vi "Show Compatibility Warnings.vi"(8 "Error In":errorcluster, 9 "Can Continue?":bool, 10 "Warnings":T1[](array[typedef]), 11 "Install LV Data":T2={"SSH Session"=refnum, "Status Log"="", "Detailed Log"="", "Credentials"={"Hostname or IP"="192.168.7.2", "Username"="root", "Password"=""}, "Target Info"={"OS Version"="", "CPU"="", "Systemd Version"="", "Internet Access"=FALSE, "Device Type"="", "LV Installed Ver"="", "LV Available Ver"="", "LV Upgrade Available"=FALSE, "Hostname"="", "NIC Info"=[]}, "Reboot Required?"=FALSE}) -> (0 "Error Out":errorcluster, 1 "Continue?":bool, 2 "Warnings":T1[](array[typedef]), 3 "Install LV Data":T2={"SSH Session"=refnum, "Status Log"="", "Detailed Log"="", "Credentials"={"Hostname or IP"="192.168.7.2", "Username"="root", "Password"=""}, "Target Info"={"OS Version"="", "CPU"="", "Systemd Version"="", "Internet Access"=FALSE, "Device Type"="", "LV Installed Ver"="", "LV Available Ver"="", "LV Upgrade Available"=FALSE, "Hostname"="", "NIC Info"=[]}, "Reboot Required?"=FALSE})   [LabVIEW 2011, in "LMH-LINX.lvlib"]
uses:
  LMH-LINX.lvlib
  Target Compatibility Warnings.ctl
  User Warning.ctl
  Install LV Data.ctl
  C:/Users/samkristoff/Desktop/Builds/2016_01_27/build/LabVIEW/vi.lib/MakerHub/LINX/Resources/Renci.SshNet.dll
  Resources/Renci.SshNet.dll
  Target Info.ctl
  NIC Info.ctl
  NIC Mode.ctl
  Status FGV States.ctl
  <vilib>/Platform/browser.llb/Open URL in Default Browser (string).vi
  <vilib>/MakerHub/Toolbox/LMH-Toolbox.lvlib
panel:
  in  "Fix It":bool
  in  "Help":bool
  out "Warning Number":string
  in  "Next":bool
  in  "Previous":bool
  out "User Warnings Dialog":T6[](array[typedef])
  out "Title":string
  out "Main Text":string
  in  "Continue":bool
  in  "Cancel":bool
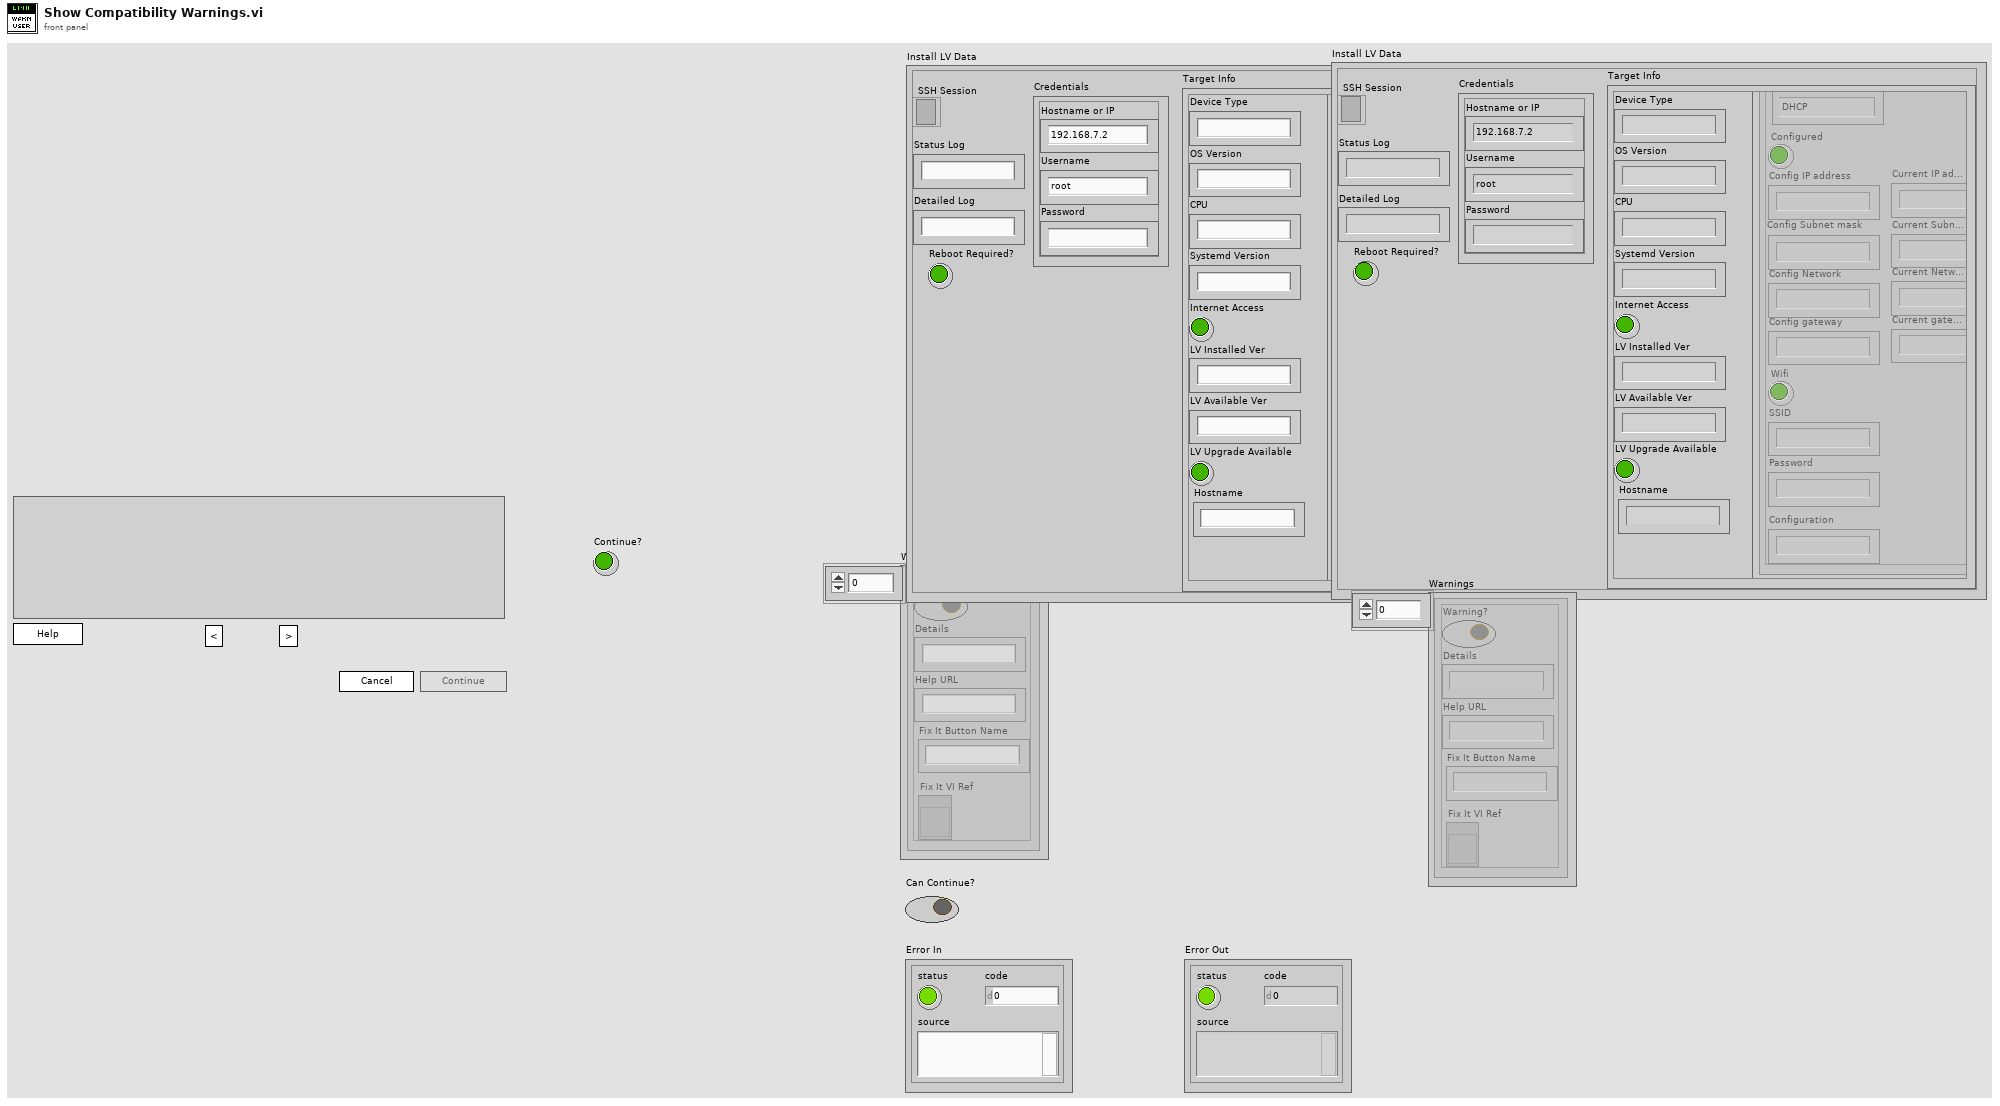
[diagram p1: front panel]
types:
  T1 = typedef "LMH-LINX.lvlib/Target Compatibility Warnings.ctl" = cluster{"Warning?":bool, "Details":string, "Help URL":string, "Fix It Button Name":string, "Fix It VI Ref":refnum<vi>}
  T2 = typedef "LMH-LINX.lvlib/Install LV Data.ctl" = cluster{"SSH Session":refnum<k24>, "Status Log":string, "Detailed Log":string, "Credentials":cluster{"Hostname or IP":string, "Username":string, "Password":string}, "Target Info":T3, "Reboot Required?":bool}
  T3 = typedef "LMH-LINX.lvlib/Target Info.ctl" = cluster{"OS Version":string, "CPU":string, "Systemd Version":string, "Internet Access":bool, "Device Type":string, "LV Installed Ver":string, "LV Available Ver":string, "LV Upgrade Available":bool, "Hostname":string, "NIC Info":T4[]}
  T4 = typedef "LMH-LINX.lvlib/NIC Info.ctl" = cluster{"Name":string, "NIC Mode":T5, "Configured":bool, "Config IP address":string, "Config Subnet mask":string, "Config Network":string, "Config gateway":string, "Wifi":bool, "SSID":string, "Password":string, "Configuration":string, "Current IP address":string, "Current Subnet mask":string, "Current gateway":string, "Current Network":string}
  T5 = typedef "LMH-LINX.lvlib/NIC Mode.ctl" = enum16{"DHCP", "Static", "Loopback"}
  T6 = typedef "LMH-LINX.lvlib/User Warning.ctl" = cluster{"Details":string, "Status":string}
  T7 = enum8{"Enabled", "Disabled", "Disabled and Grayed Out"}
  T8 = typedef "LMH-LINX.lvlib/Status FGV States.ctl" = enum16{"Init", "Append", "Append History Only", "Set", "Get"}
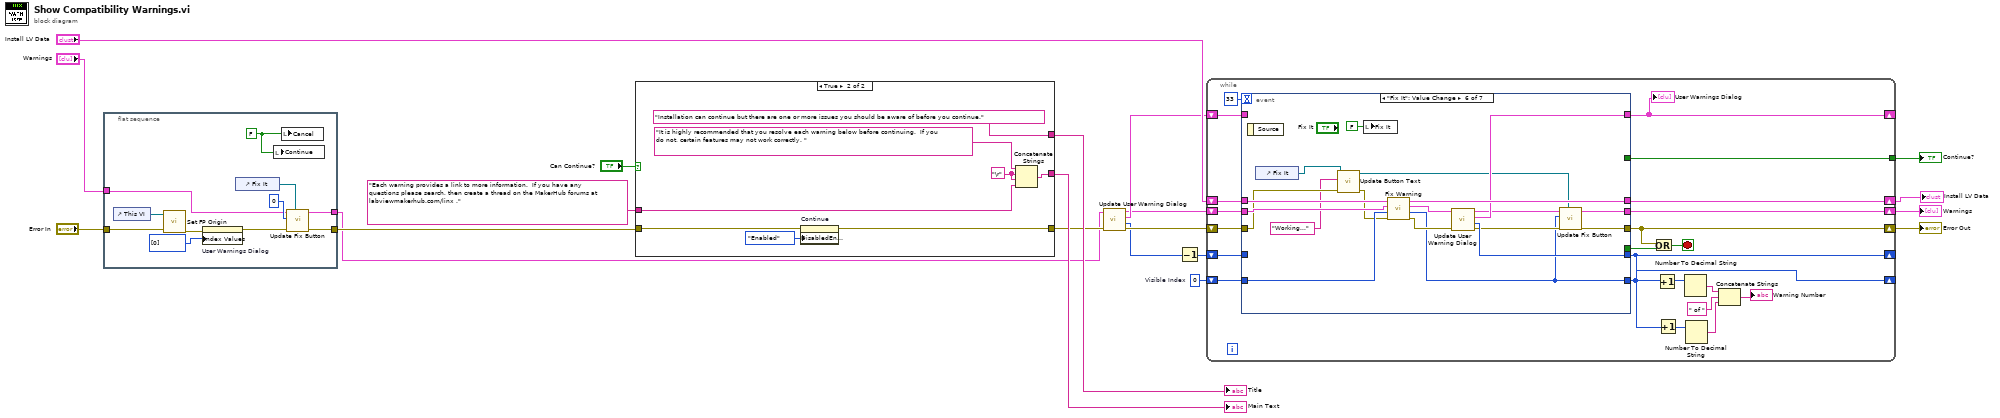
[diagram p0: block diagram]
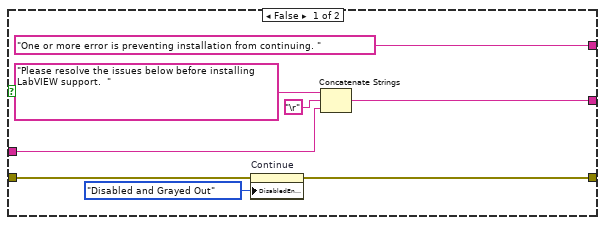
[diagram p2: hidden frame]
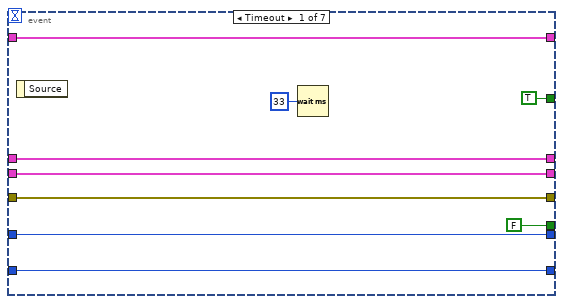
[diagram p3: hidden frame]
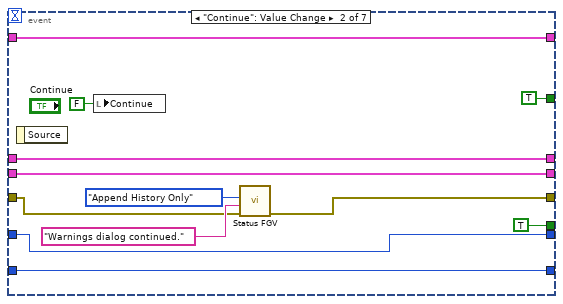
[diagram p4: hidden frame]
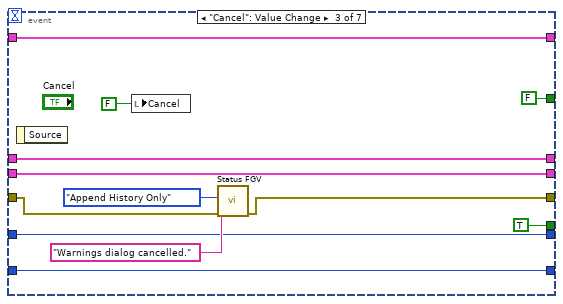
[diagram p5: hidden frame]
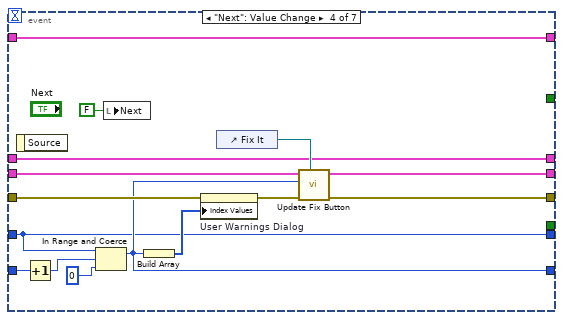
[diagram p6: hidden frame]
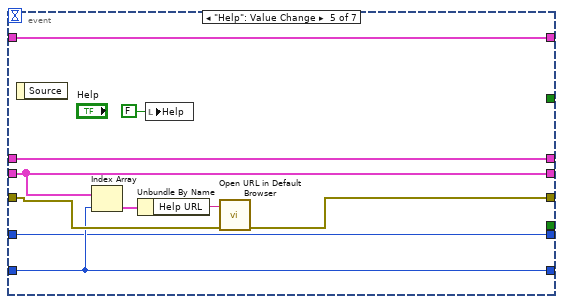
[diagram p7: hidden frame]
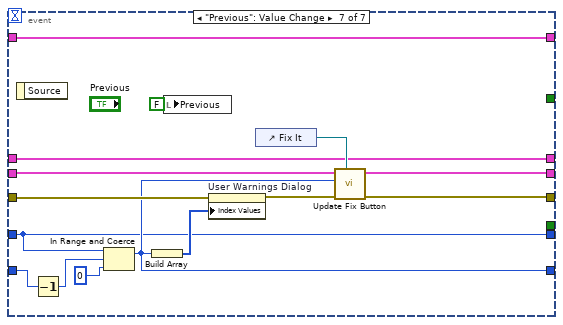
[diagram p8: hidden frame]
diagram:
  w10 = 0  # Visible Index
  n1 = flat-sequence {
    tunnel: [w26] -> w15
    tunnel: "Error In" -> [w29]
    tunnel: "Warnings" -> [w22]
    tunnel: [w21] -> w6
    frame #0 {
      w31 = FALSE ("Cancel")
      n2 = control-ref of="This VI"() -> (w27:refnum<vi>)
      n3 = call <vilib>:"Set FP Origin.vi"("Error In"=w29, "VI Ref"=w27) -> ("Error Out"=w28:errorcluster)  [unwired: 9 in]
      n4 = property on="User Warnings Dialog" class="Arr (strict)"(error in=w28, "Index Values"=u32[] [0]) -> (error out=w25:errorcluster)  [unwired: 1 in, 1 out]
      n5 = control-ref of="Fix It"() -> (w24:refnum<vi>)
      n6 = local write "Continue"(w31) -> ()
      n7 = local write "Cancel"(w31) -> ()
      n8 = call "Update Fix Button.vi"("Fix It Button Ref"=w24, "Error In"=w25, "Warning Index"=0, "Warnings"=w22) -> ("Error Out"=w26:errorcluster, "Warnings"=w21:T1[])  [unwired: 6 in]
    }
  }
  n9 = case shown="True" "Can Continue?" {
    tunnel: [w36 w46] -> w19
    tunnel: "Each warning provides a link to more information.  If you have any questions please search, then create a thread on the MakerHub forums at labviewmakerhub.com/linx ." ("Main Text") -> [w37 w41]
    tunnel: ["One or more error is preventing installation from continuing. " ("Main Text") "Installation can continue but there are one or more issues you should be aware of before you continue."] -> w17
    tunnel: [w32 w43] -> w16
    tunnel: w15 -> [w33 w44]
    frame False {
      n10 = property on="Continue" class="Bool (strict)"(error in=w33, "DisabledEnum"=T7."Disabled and Grayed Out" ("Disabled")) -> (error out=w32:errorcluster)  [unwired: 1 in, 1 out]
      n11 = Concatenate Strings("Please resolve the issues below before installing LabVIEW support.  " ("Main Text"), "\r", w37) -> (w36:string)
    }
    frame True {
      w40 = "\r"
      n12 = property on="Continue" class="Bool (strict)"(error in=w44, "DisabledEnum"=T7."Enabled" ("Disabled")) -> (error out=w43:errorcluster)  [unwired: 1 in, 1 out]
      n13 = Concatenate Strings("It is highly recommended that you resolve each warning below before continuing.  If you do not, certain features may not work correctly. " ("Main Text"), w40, w40, w41) -> (w46:string)
    }
  }
  "Main Text" <- w19
  "Title" <- w17
  n14 = call "Update User Warning Dialog.vi"("Error In"=w16, "Warnings"=w6) -> ("Error Out"=w13:errorcluster, "Num Warnings"=w2:i32, "User Warnings"=w3:T6[], "Warnings"=w1:T1[])  [unwired: 6 in]
  n15 = Decrement(x=w2) -> (x-1=w9:i32)
  n16 = while {
    shift-right: [w67] -> w12
    shift-left: w13 -> [w69]
    tunnel: [w65] -> w11
    shift-right: [w57] -> _
    shift-left: w10 -> [w63]
    shift-right: [w55] -> w8
    shift-left: w1 -> [w62]
    shift-right: [w53] -> w4
    shift-left: "Install LV Data" -> [w54]
    shift-right: [w48] -> _
    shift-left: w3 -> [w52]
    shift-right: [w50] -> _
    shift-left: w9 -> [w64]
    stop <- w66 stop-if-true
    n17 = event shown="[5] \"Fix It\": Value Change" {
      selector: _ -> [_ _ _ _ _ _ _]
      dyn-events: _ -> [_ _ _ _ _ _ _]
      timeout: 33 -> [_ _ _ _ _ _ _]
      tunnel: [w77 w84 w97 w110 w124 w136 w149] -> w67
      tunnel: w69 -> [w77 w83 w98 w112 w125 w130 w156]
      tunnel: [FALSE TRUE TRUE _ _ _ _] -> w68
      tunnel: [TRUE TRUE FALSE _ _ _ _] -> w65
      tunnel: w64 -> [w71 w80 w92 w103 w119 _ w148]
      tunnel: w63 -> [w75 w87 w99 w115 w122 w139 w159]
      tunnel: [w75 w87 w99 w108 w122 w133 w152] -> w57
      tunnel: w62 -> [w73 w82 w94 w109 w121 w143 w153]
      tunnel: [w73 w82 w94 w107 w121 w134 w150] -> w55
      tunnel: w54 -> [w72 w81 w93 w105 w120 w145 w151]
      tunnel: [w72 w81 w93 w105 w120 w144 w151] -> w53
      tunnel: [w70 w79 w91 w104 w118 w140 w147] -> w48
      tunnel: w52 -> [w70 w79 w91 w104 w118 _ w147]
      tunnel: [w71 w80 w92 w103 w119 w138 w148] -> w50
      event Timeout {
        n18 = event-data() -> ()  [unwired: 1 in, 1 out]
        n19 = Wait (ms)(milliseconds to wait=u32 33) -> ()  [unwired: 1 out]
      }
      event "Continue": Value Change {
        n20 = event-data() -> ()  [unwired: 1 in, 1 out]
        n21 = local write "Continue"(FALSE ("Continue")) -> ()
        n22 = call "Status FGV.vi"("Error In"=w83, "Status"="Warnings dialog continued.", "Status FGV State"=Status_FGV_States."Append History Only") -> ("Error Out"=w84:errorcluster)  [unwired: 6 in, 2 out]
      }
      event "Cancel": Value Change {
        n23 = event-data() -> ()  [unwired: 1 in, 1 out]
        n24 = local write "Cancel"(FALSE ("Continue")) -> ()
        n25 = call "Status FGV.vi"("Error In"=w98, "Status"="Warnings dialog cancelled.", "Status FGV State"=Status_FGV_States."Append History Only") -> ("Error Out"=w97:errorcluster)  [unwired: 6 in, 2 out]
      }
      event "Next": Value Change {
        n26 = event-data() -> ()  [unwired: 1 in, 1 out]
        n27 = Increment(x=w115) -> (x+1=w114:i32)
        n28 = In Range and Coerce(upper limit=w103, x=w114, lower limit=0) -> (coerced(x)=w108:i32)  [unwired: 1 out]
        n29 = local write "Next"(FALSE ("Next")) -> ()
        n30 = Build Array(w108) -> (w113:i32[])
        n31 = property on="User Warnings Dialog" class="Arr (strict)"(error in=w112, "Index Values"=w113) -> (error out=w111:errorcluster)  [unwired: 1 in, 1 out]
        n32 = control-ref of="Fix It"() -> (w106:refnum<vi>)
        n33 = call "Update Fix Button.vi"("Fix It Button Ref"=w106, "Error In"=w111, "Warning Index"=w108, "Warnings"=w109) -> ("Error Out"=w110:errorcluster, "Warnings"=w107:T1[])  [unwired: 6 in]
      }
      event "Help": Value Change {
        n34 = event-data() -> ()  [unwired: 1 in, 1 out]
        n35 = Index Array(array=w121, index=w122) -> (element=w126:T1)
        n36 = Unbundle By Name(w126) -> ("Help URL"=w123:string)
        n37 = local write "Help"(FALSE ("Help")) -> ()
        n38 = call-poly <vilib>:"Open URL in Default Browser.vi"("error in (no error)"=w125, "URL"=w123) -> ("error out"=w124:errorcluster)  [unwired: 4 in, 1 out]
      }
      event "Fix It": Value Change {
        n39 = event-data() -> ()  [unwired: 1 in, 1 out]
        n40 = control-ref of="Fix It"() -> (w131:refnum<vi>)
        n41 = call "Update Button Text.vi"("Error In"=w130, "Button Text"="Working...", "Button Ref"=w131) -> ("Error Out"=w132:errorcluster, "Buffon Ref"=w129:refnum<vi>)  [unwired: 7 in]
        n42 = local write "Fix It"(FALSE ("Fix It")) -> ()
        n43 = call "Fix Warning.vi"("Error In"=w132, "Warning Index"=w139, "Warnings"=w143, "Install LV Data in"=w145) -> ("Error Out"=w141:errorcluster, "Visible Index"=w133:i32, "Warnings"=w142:T1[], "Install LV Data out"=w144:T2)  [unwired: 4 in]
        n44 = call "Update User Warning Dialog.vi"("Error In"=w141, "Warnings"=w142) -> ("Error Out"=w137:errorcluster, "Num Warnings"=w138:i32, "User Warnings"=w140:T6[], "Warnings"=w135:T1[])  [unwired: 6 in]
        n45 = call "Update Fix Button.vi"("Fix It Button Ref"=w129, "Error In"=w137, "Warning Index"=w133, "Warnings"=w135) -> ("Error Out"=w136:errorcluster, "Warnings"=w134:T1[])  [unwired: 6 in]
      }
      event "Previous": Value Change {
        n46 = event-data() -> ()  [unwired: 1 in, 1 out]
        n47 = Decrement(x=w159) -> (x-1=w158:i32)
        n48 = In Range and Coerce(upper limit=w148, x=w158, lower limit=0) -> (coerced(x)=w152:i32)  [unwired: 1 out]
        n49 = Build Array(w152) -> (w157:i32[])
        n50 = local write "Previous"(FALSE ("Next")) -> ()
        n51 = property on="User Warnings Dialog" class="Arr (strict)"(error in=w156, "Index Values"=w157) -> (error out=w154:errorcluster)  [unwired: 1 in, 1 out]
        n52 = control-ref of="Fix It"() -> (w155:refnum<vi>)
        n53 = call "Update Fix Button.vi"("Fix It Button Ref"=w155, "Error In"=w154, "Warning Index"=w152, "Warnings"=w153) -> ("Error Out"=w149:errorcluster, "Warnings"=w150:T1[])  [unwired: 6 in]
      }
    }
    "User Warnings Dialog" <- w48
    n54 = Or(x=w67, y=w68) -> (x .or. y?=w66:bool)
    n55 = Increment(x=w57) -> (x+1=w58:i32)
    n56 = Increment(x=w50) -> (x+1=w49:i32)
    n57 = Number To Decimal String(number=w58) -> (decimal integer string=w61:string)  [unwired: 1 in]
    n58 = Number To Decimal String(number=w49) -> (decimal integer string=w51:string)  [unwired: 1 in]
    n59 = Concatenate Strings(w61, " of ", w51) -> (→"Warning Number":string)
  }
  "Error Out" <- w12
  "Continue?" <- w11
  "Install LV Data" <- w4
  "Warnings" <- w8
